vi "Send Throttle Signal.vi"(9 "Requested Torque (Nm)":dbl format="%#_13g", 10 "CAN Offset":u32=160 format="%x", 11 "CANTXQueueIn":T1) -> (3 "CANTXQueueOut":T1)   [LabVIEW 2015]
uses:
  TX Library/CAN Message Queue.ctl
  TX Library/CAN Message.ctl
  <vilib>/RioEmbeddedCAN/RioEmbeddedCAN.llb/CANFrameControl.ctl
panel:
  out "(hi.lo)":i16
  in  "Direction":u8=1
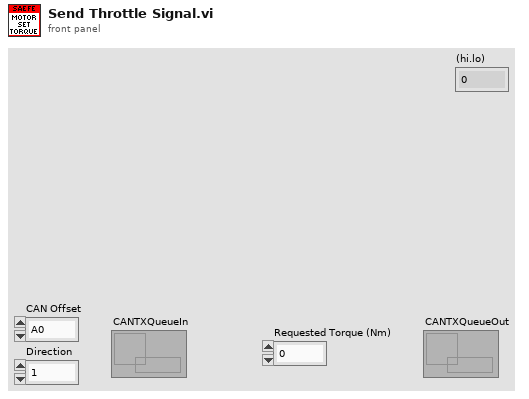
[diagram p1: front panel]
types:
  T1 = typedef "CAN Message Queue.ctl" = refnum<k33>
  T2 = typedef "CANFrameControl.ctl" = cluster{"identifier":u32, "extended?":bool, "type":u8, "payload":u8[]}
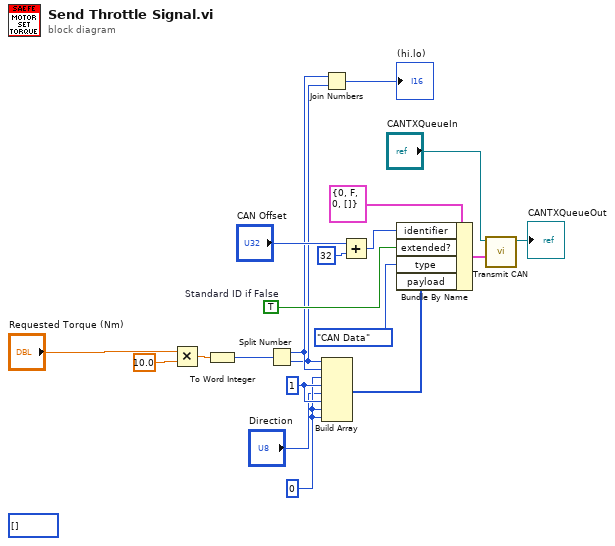
[diagram p0: block diagram]
diagram:
  (unwired) u8[] []
  w11 = u8 0 ("element")
  w12 = u8 1 ("element")
  w18 = TRUE  # Standard ID if False
  n1 = Multiply(x="Requested Torque (Nm)", y=10.0) -> (x*y=w8:dbl)
  n2 = To Word Integer(number=w8) -> (16bit integer=w4:i16)
  n3 = Split Number(x=w4) -> (hi(x)=w3:u8, lo(x)=w2:u8)
  n4 = Join Numbers(hi=w3, lo=w2) -> ((hi.lo)=→"(hi.lo)":u16)
  n5 = Build Array(w2, w3, w11, w12, "Direction", w12, w11, w11) -> (w16:u8[])
  n6 = Add(x="CAN Offset", y=u32 32 ("identifier")) -> (x+y=w14:u32)
  n7 = Bundle By Name(cluster=T2 {"identifier"=0, "extended?"=FALSE, "type"=0, "payload"=[]} ("CAN frame"), "identifier"=w14, "extended?"=w18, "type"=enum8{"CAN Data", "CAN Remote"}."CAN Data", "payload"=w16) -> (w7:T2)
  n8 = call "Transmit CAN.vi"("CAN Queue"="CANTXQueueIn", "CAN frame"=w7) -> ("CAN Queue Out"=→"CANTXQueueOut":T1)  [unwired: 8 in]
